vi "p03 posicion de pelota.vi"() -> ()   [LabVIEW 2013]
uses:
  <vilib>/Math Plots/3D Math Plots/3D Mesh/3D Mesh Datatype/3D Mesh Datatype.lvclass
  <vilib>/Math Plots/3D Math Plots/3D Mesh/3D Mesh Datatype/Public/Plot Helper (Matrix).vi
  <vilib>/Math Plots/3D Math Plots/3D Mesh/3D Mesh XCtrl/3D Mesh.xctl
panel:
  out "x/y 2":dbl
  out "x/y":dbl
  out "Waveform Chart 2":dbl[](graph)
  out "Waveform Chart":dbl[](graph)
  out "3D Mesh":refnum<class "3D Plot Datatype.lvclass">[](xcontrol)
  in  "Slide":dbl(slide) scale=0.0..255.0
  in  "path to BMP file":path
  out "new picture":picture
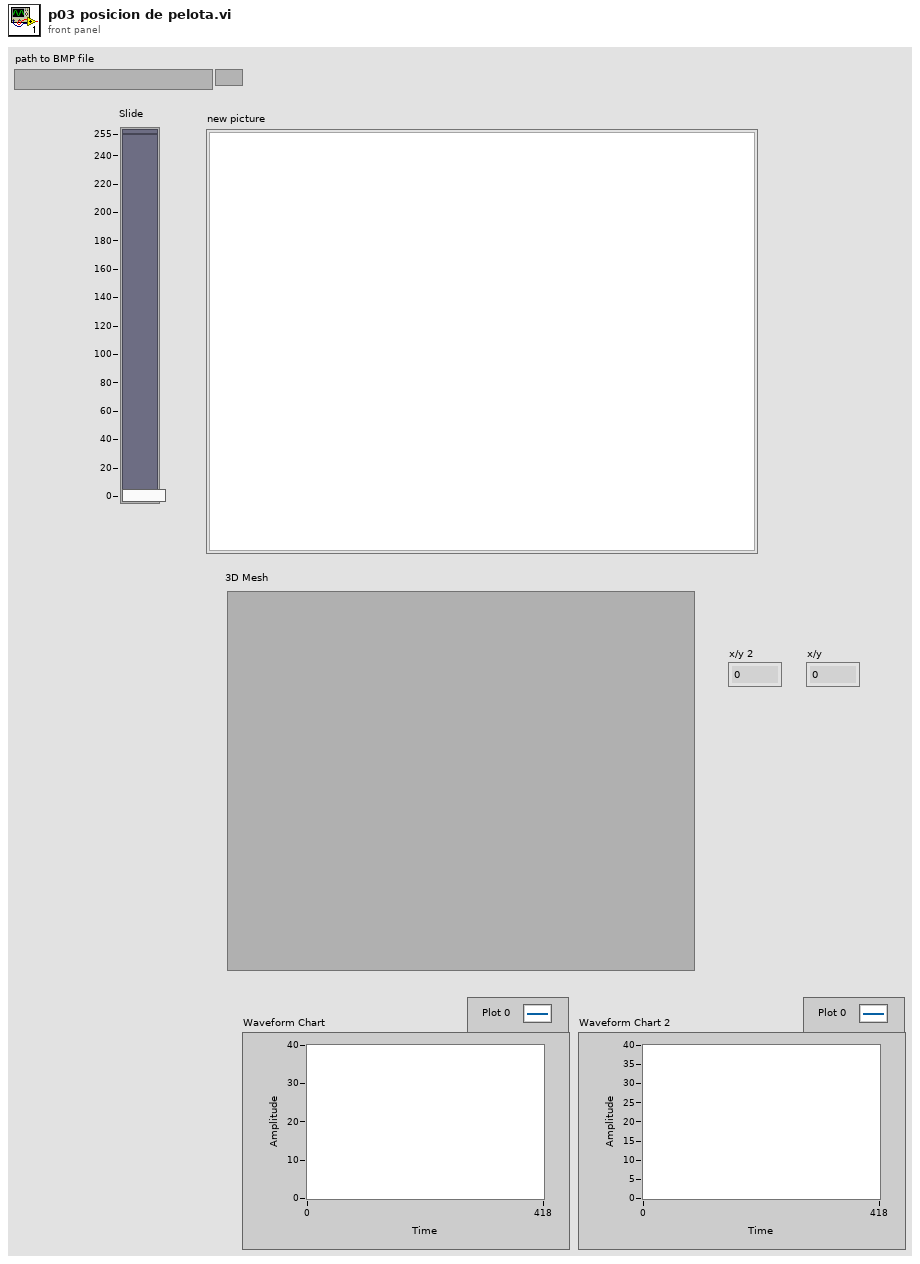
[diagram p1: front panel]
types:
  T1 = typedef "imagedata.ctl" = cluster{"image type":i32, "image depth":i32, "image":u8[], "mask":u8[], "colors":u32[], "Rectangle":cluster{"left":i16, "top":i16, "right":i16, "bottom":i16}}
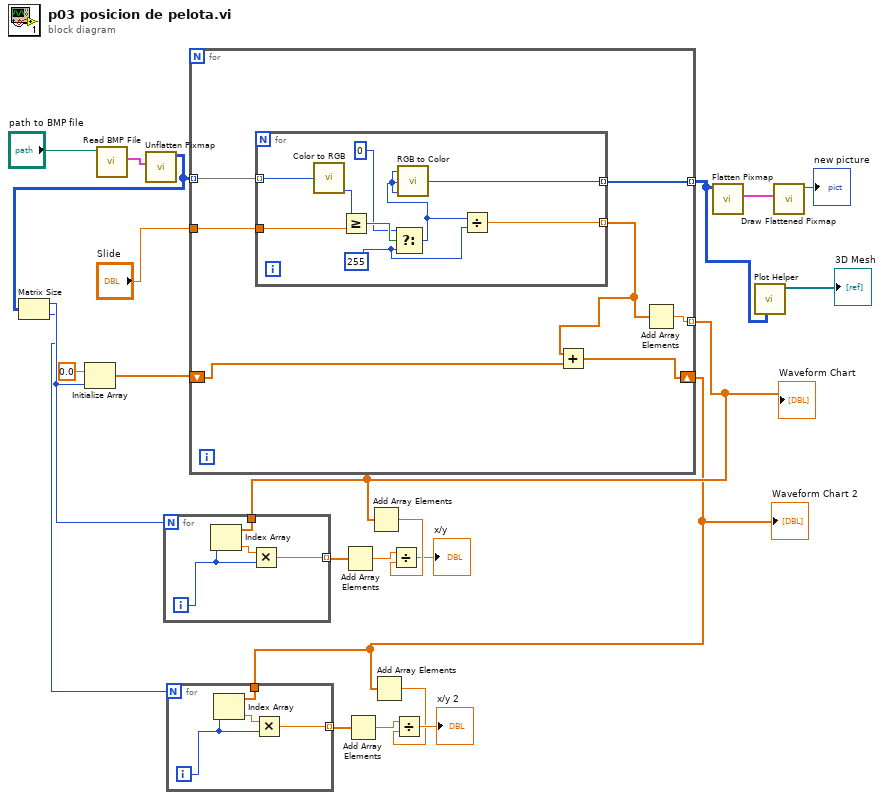
[diagram p0: block diagram]
diagram:
  n1 = call <vilib>:"Read BMP File.vi"("path to BMP file"="path to BMP file") -> ("image data"=w15:T1)  [unwired: 8 in, 2 out]
  n2 = call <vilib>:"Unflatten Pixmap.vi"("image data"=w15) -> ("24-bit pixmap"=w14:u32[][])  [unwired: 4 in, 6 out]
  n3 = Matrix Size(0:w14) -> (1:w12:i32, 2:w1:i32)
  n4 = Initialize Array(0.0 ("element"), w12) -> (w13:dbl[])
  n5 = for {
    tunnel: w14 -> [w29] mode=indexing
    tunnel: [w26] -> w17 mode=indexing
    tunnel: "Slide" -> [w28]
    tunnel: [w27] -> w9 mode=indexing
    shift-right: [w24] -> w2
    shift-left: w13 -> [w25]
    n6 = for {
      tunnel: w29 -> [w38] mode=indexing
      tunnel: [w33] -> w26 mode=indexing
      tunnel: w28 -> [w37]
      tunnel: [w31] -> w23 mode=indexing
      w32 = 255
      n7 = call <vilib>:"Color to RGB.vi"("Color"=w38) -> ("B"=w34:u8)  [unwired: 3 out]
      n8 = Greater Or Equal?(x=w34, y=w37) -> (x >= y?=w36:bool)
      n9 = Select(t=0, s=w36, f=w32) -> (s? t:f=w30:i32)
      n10 = call <vilib>:"RGB to Color.vi"("B"=w30, "G"=w30, "R"=w30) -> ("Color"=w33:u32)
      n11 = Divide(x=w30, y=w32) -> (x/y=w31:dbl)
    }
    n12 = Add(x=w23, y=w25) -> (x+y=w24:dbl[])
    n13 = Add Array Elements(numeric array=w23) -> (sum=w27:dbl)
  }
  "Waveform Chart" <- w9
  "Waveform Chart 2" <- w2
  n14 = for {
    N: w12 -> [_]
    tunnel: w9 -> [w41]
    tunnel: [w42] -> w11 mode=indexing
    i -> [w40]
    n15 = Index Array(array=w41, index=w40) -> (element=w39:dbl)
    n16 = Multiply(x=w39, y=w40) -> (x*y=w42:dbl)
  }
  n17 = for {
    N: w1 -> [_]
    tunnel: w2 -> [w45]
    tunnel: [w46] -> w3 mode=indexing
    i -> [w44]
    n18 = Index Array(array=w45, index=w44) -> (element=w43:dbl)
    n19 = Multiply(x=w43, y=w44) -> (x*y=w46:dbl)
  }
  n20 = Add Array Elements(numeric array=w11) -> (sum=w10:dbl)
  n21 = Add Array Elements(numeric array=w3) -> (sum=w4:dbl)
  n22 = Add Array Elements(numeric array=w9) -> (sum=w8:dbl)
  n23 = Add Array Elements(numeric array=w2) -> (sum=w5:dbl)
  n24 = Divide(x=w10, y=w8) -> (x/y=→"x/y":dbl)
  n25 = Divide(x=w4, y=w5) -> (x/y=→"x/y 2":dbl)
  n26 = call <vilib>:"Flatten Pixmap.vi"("24-bit pixmap"=w17) -> ("image data"=w22:T1)  [unwired: 10 in]
  n27 = call-poly <vilib>:"Plot Helper.vi"("z matrix"=w17) -> ("3D Plot lvclass Array out"=→"3D Mesh":refnum<class "3D Plot Datatype.lvclass">[])  [unwired: 5 in, 5 out]
  n28 = call <vilib>:"Draw Flattened Pixmap.vi"("image data"=w22) -> ("new picture"=→"new picture":picture)  [unwired: 8 in]
